vi "Do Something.vi"(8 "error in (no error)":errorcluster, 10 "Bytes to Read":i32, 11 "Inst.Magneto in":refnum<class "Inst.Magneto.lvclass">) -> (0 "error out":errorcluster, 3 "Inst.Magneto out":refnum<class "Inst.Magneto.lvclass">)   [LabVIEW 2019, in "Inst.Magneto.lvclass"]
uses:
  Inst.Magneto.lvclass
  67792bfe-8e2c-4879-abc2-cb448bcec168.vi
  Typedefs/Inst.Magneto.Commands--Enum.ctl
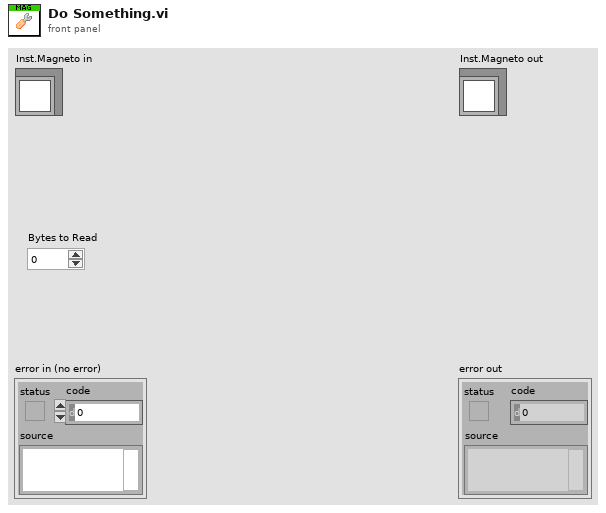
[diagram p1: front panel]
types:
  T1 = typedef "Inst.Magneto.lvclass/Inst.Magneto.Commands--Enum.ctl" = enum16{"Clear Values"}
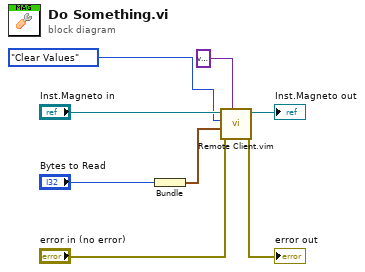
[diagram p0: block diagram]
diagram:
  n1 = Bundle("Bytes to Read"="Bytes to Read") -> (w3:cluster{"Bytes to Read":i32})  [unwired: 1 in]
  n2 = call "Remote Client.vim"("Data Out type"=variant, "error in (no error)"="error in (no error)", "params"=w3, "method"=Inst.Magneto.Commands--Enum."Clear Values" ("Commands"), "Instrument in"="Inst.Magneto in") -> ("error out"=→"error out":errorcluster, "Instrument out"=→"Inst.Magneto out":refnum<class "Inst.Magneto.lvclass">)  [unwired: 3 in, 2 out]
